vi "JSON type.vi"(10 "Offset":i32, 11 "JSON":string) -> (2 "Starting Offset":i32, 3 "JSON Value Type":T1)   [LabVIEW 2015, in "JSONtext.lvlib"]
doc: "Determines the type of a JSON Value (object, array, string, number, true, false, or null)\n\n\"Offset\" should point to the start of the JSON Value, or to whitespace in front of the Value.\n\nThis function does not do a full validation of the Value, but instead identifies it only from its start (so, for example, something starting with \"{\" will be identified as a JSON Object)."
uses:
  JSONtext.lvlib
  JSON Value Type.ctl
  Parsing State.ctl
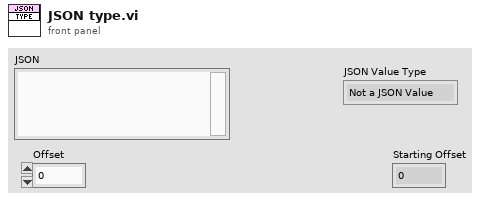
[diagram p1: front panel]
types:
  T1 = typedef "JSON Value Type.ctl" = enum16{"Not a JSON Value", "JSON Object", "JSON Array", "String", "Number", "true", "false", "null"}
  T2 = typedef "JSONtext.lvlib/Parsing State.ctl" = enum16{"Parser Error", "Object", "Array", "String", "Number/Other", "Leading Whitespace", "Object end", "Array end", "Value end"}
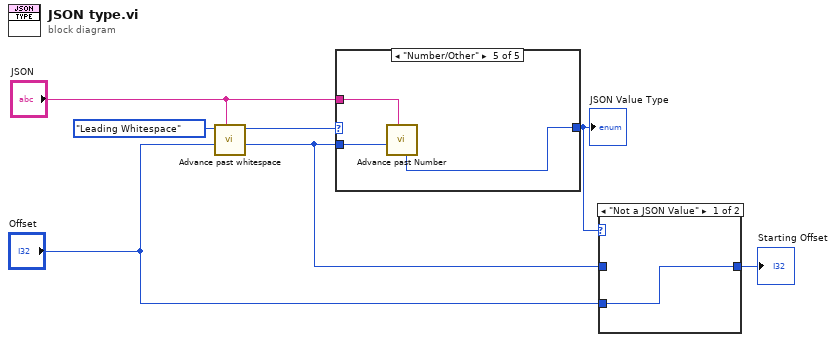
[diagram p0: block diagram]
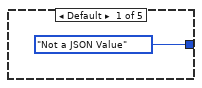
[diagram p2: hidden frame]
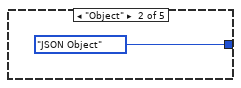
[diagram p3: hidden frame]
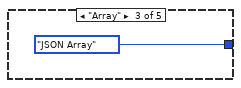
[diagram p4: hidden frame]
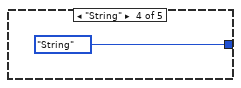
[diagram p5: hidden frame]
diagram:
  n1 = call "Advance past whitespace.vi"("JSON"="JSON", "Offset"="Offset", "Parser State in"=Parsing_State."Leading Whitespace") -> ("Offset of first non-whitespace"=w2:i32, "Parser State"=w6:T2)  [unwired: 7 in]
  n2 = case shown="\"Number/Other\"" w6 {
    tunnel: [JSON_Value_Type."Not a JSON Value" JSON_Value_Type."JSON Object" JSON_Value_Type."JSON Array" JSON_Value_Type."String" w12] -> w4
    tunnel: "JSON" -> [_ _ _ _ w13]
    tunnel: w2 -> [_ _ _ _ w14]
    frame Default {
    }
    frame "Object" {
    }
    frame "Array" {
    }
    frame "String" {
    }
    frame "Number/Other" {
      n3 = call "Advance past Number.vi"("JSON"=w13, "Offset (0)"=w14) -> ("JSON Value Type"=w12:T1)  [unwired: 6 in, 3 out]
    }
  }
  "JSON Value Type" <- w4
  n4 = case shown="\"Not a JSON Value\"" w4 {
    tunnel: [w15 w16] -> w3
    tunnel: w2 -> [_ w16]
    tunnel: "Offset" -> [w15 _]
    frame "Not a JSON Value" {
    }
    frame Default {
    }
  }
  "Starting Offset" <- w3
